vi "Get 420 State.vi"(0 "VISA session":refnum<visa-resource-name>="GPIB0::22::INSTR") -> (1 "State":T1(ring), 2 "Switch Heater Voltage":dbl format="%.2f", 3 "dup VISA session":refnum<visa-resource-name>, 4 "Switch Heater":bool, 5 "Switch heater \nconfirmed":bool, 6 "Switch Heater Error":bool)   [LabVIEW 2020]
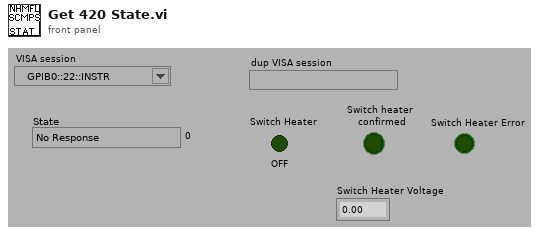
[diagram p1: front panel]
types:
  T1 = enum16{"No Response", "Ramping to programmed field ", "Holding at programmed field", "Paused", "Ramp Manual Up", "Ramp Manual Down", "Ramping to Zero", "QUENCH", "Heating Persistence Switch", "At Zero Current"}
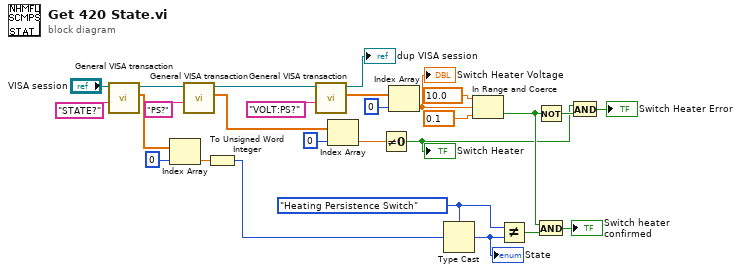
[diagram p0: block diagram]
diagram:
  w1 = T1."Heating Persistence Switch" ("State")
  n1 = call "General VISA transaction.vi"("Command String"="STATE?", "VISA Session"="VISA session") -> ("Measurement"=w25:dbl[], "dup VISA Session"=w22:refnum<visa-resource-name>)  [unwired: 4 in, 4 out]
  n2 = Index Array(array=w25, index=0) -> (element=w23:dbl)
  n3 = call "General VISA transaction.vi"("Command String"="PS?", "VISA Session"=w22) -> ("Measurement"=w20:dbl[], "dup VISA Session"=w17:refnum<visa-resource-name>)  [unwired: 4 in, 4 out]
  n4 = To Unsigned Word Integer(number=w23) -> (unsigned 16bit integer=w3:u16)
  n5 = call "General VISA transaction.vi"("Command String"="VOLT:PS?", "VISA Session"=w17) -> ("Measurement"=w15:dbl[], "dup VISA Session"=→"dup VISA session":refnum<visa-resource-name>)  [unwired: 4 in, 4 out]
  n6 = Index Array(array=w20, index=0) -> (element=w18:dbl)
  n7 = Not Equal To 0?(x=w18) -> (x != 0?=w5:bool)
  "Switch Heater" <- w5
  n8 = Index Array(array=w15, index=0) -> (element=w12:dbl)
  "Switch Heater Voltage" <- w12
  n9 = Type Cast(type=w1, x=w3) -> (*(type *) &x=w2:T1)
  "State" <- w2
  n10 = In Range and Coerce(upper limit=10.0 ("y"), x=w12, lower limit=0.1) -> (In Range?=w7:bool)  [unwired: 1 out]
  n11 = Not Equal?(x=w1, y=w2) -> (x != y?=w9:bool)
  n12 = Not(x=w7) -> (.not. x?=w6:bool)
  n13 = And(x=w7, y=w9) -> (x .and. y?=→"Switch heater \nconfirmed":bool)
  n14 = And(x=w5, y=w6) -> (x .and. y?=→"Switch Heater Error":bool)
